vi "clearpath_write_serial.vi"(2 "queue in":refnum<queue>, 3 "error in":errorcluster, 4 "VISA resource name in":refnum<visa-resource-name>) -> (0 "error out":errorcluster, 1 "VISA resource name out":refnum<visa-resource-name>)   [LabVIEW 2012, in "clearpath_interface.lvlib"]
doc: "Dequeues valid CCP messages from the provided queue and transmits them to the connected Clearpath platform."
uses:
  IGVC/Clearpath/Husky 2011/Teleop Robotics Project Folder/Husky/vi/clearpath_interface.lvlib
panel:
  out "TX String":string
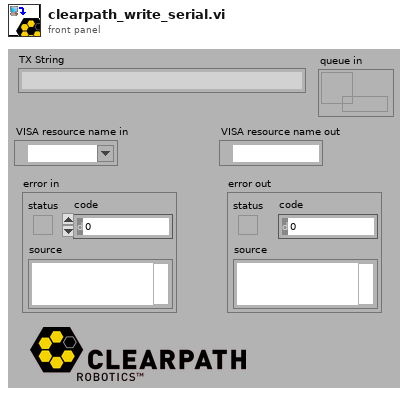
[diagram p1: front panel]
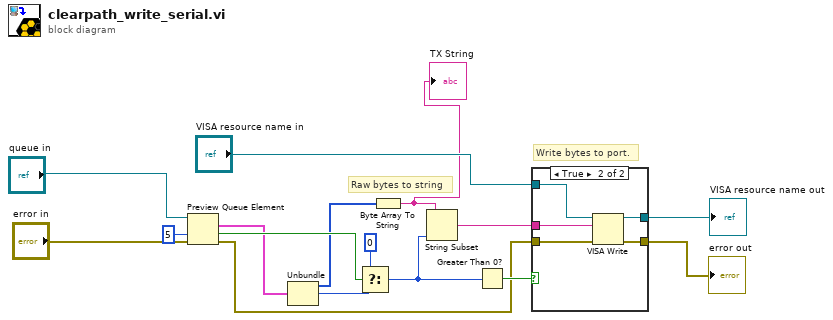
[diagram p0: block diagram]
diagram:
  # "Write bytes to port."
  # "Raw bytes to string"
  n1 = Preview Queue Element(queue="queue in", timeout in ms (-1)=5, error in (no error)="error in") -> (element=w8:cluster{i32[], i32, i32}, timed out?=w12:bool, error out=w3:errorcluster)  [unwired: 1 out]
  n2 = Unbundle(w8) -> (w10:i32[], w13:i32)  [unwired: 1 out]
  n3 = Select(t=0, s=w12, f=w13) -> (s? t:f=w16:i32)
  n4 = Byte Array To String(unsigned byte array=w10) -> (string=w2:string)
  "TX String" <- w2
  n5 = String Subset(string=w2, length (rest)=w16) -> (substring=w11:string)  [unwired: 1 in]
  n6 = Greater Than 0?(x=w16) -> (x > 0?=w15:bool)
  n7 = case shown="True" w15 {
    tunnel: "VISA resource name in" -> [w18 w21]
    tunnel: [w18 w23] -> w7
    tunnel: w3 -> [w17 w20]
    tunnel: [w17 w22] -> w5
    tunnel: w11 -> [_ w19]
    frame False {
    }
    frame True {
      n8 = VISA Write(VISA resource name=w21, write buffer=w19, error in (no error)=w20) -> (VISA resource name out=w23:refnum<visa-resource-name>, error out=w22:errorcluster)  [unwired: 1 out]
    }
  }
  "error out" <- w5
  "VISA resource name out" <- w7
